vi "MALT Get Counter.vi"(8 "error in":errorcluster, 9 "Port":i32=1, 10 "Address":i32=3, 11 "FamilyCode":T1=enum."MALT132") -> (0 "error out":errorcluster, 3 "Value":u32)   [LabVIEW 2018, in "AltonTech MALT200817.lvlib"]
uses:
  <instrlib>/AltonTech MALT/AltonTech MALT200817.lvlib
  <instrlib>/AltonTech MALT/Public/Types/MALT CardTypes.ctl
  <instrlib>/AltonTech MALT/Private/Global/MALT Global.vi
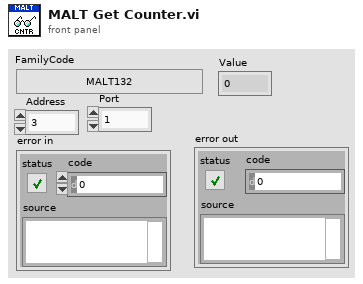
[diagram p1: front panel]
types:
  T1 = typedef "AltonTech MALT200817.lvlib/MALT CardTypes.ctl" = enum32{"-", "YAV90832", "YAV904X8", "MALT132", "YAV91616", "YAV90PIN", "YAV90096", "YAV90HVT", "YAV90CLR", "YAV90128", "YAV90PNE", "YAVCANCON", "YAV91775", "YAV90XXX", "YAV90MMU", "H730050", "H710060", "H710061", "YAV90304", "MMI", "YAV90060", "MALT160T", "YAV90059", "Not Defined"}
  T2 = cluster{"Timeout":i32, "CAN Response Delay":i32, "Connection ID":refnum<k5>}
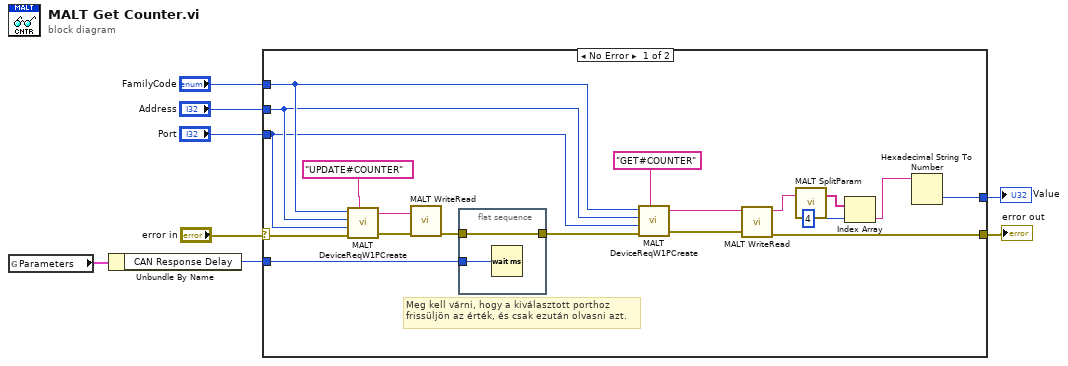
[diagram p0: block diagram]
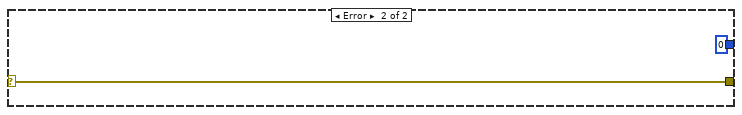
[diagram p2: hidden frame]
diagram:
  n1 = global read "MALT Global.vi" "Parameters"() -> (w3:T2)
  n2 = Unbundle By Name(w3) -> ("CAN Response Delay"=w2:i32)
  n3 = case shown="No Error" "error in" {
    selector: "error in" -> [w9 w31]
    tunnel: "FamilyCode" -> [w23 _]
    tunnel: "Address" -> [w22 _]
    tunnel: "Port" -> [w21 _]
    tunnel: [w12 w31] -> w5
    tunnel: [w11 u32 0] -> w4
    tunnel: w2 -> [w10 _]
    frame No Error {
      # "Meg kell várni, hogy a kiválasztott porthoz \nfrissüljön az érték, és csak ezután olvasni azt."
      n4 = call <instrlib>:"MALT DeviceReqW1PCreate.vi"("FamilyCode"=w23, "Address"=w22, "Param1"=w21, "error in"=w9, "Cmd"="UPDATE#COUNTER") -> ("Request"=w25:string, "error out"=w26:errorcluster)  [unwired: 1 in]
      n5 = call <instrlib>:"MALT WriteRead.vi"("error in"=w26, "Request"=w25) -> ("error out"=w19:errorcluster)  [unwired: 8 in, 1 out]
      n6 = flat-sequence {
        tunnel: [w29] -> w20
        tunnel: w19 -> [w29]
        tunnel: w10 -> [w28]
        frame #0 {
          n7 = Wait (ms)(milliseconds to wait=w28) -> ()  [unwired: 1 out]
        }
      }
      n8 = call <instrlib>:"MALT DeviceReqW1PCreate.vi"("FamilyCode"=w23, "Address"=w22, "Param1"=w21, "error in"=w20, "Cmd"="GET#COUNTER") -> ("Request"=w13:string, "error out"=w14:errorcluster)  [unwired: 1 in]
      n9 = call <instrlib>:"MALT WriteRead.vi"("error in"=w14, "Request"=w13) -> ("error out"=w12:errorcluster, "Response"=w17:string)  [unwired: 8 in]
      n10 = call <instrlib>:"MALT SplitParam.vi"("Line"=w17) -> ("Items"=w16:string[])  [unwired: 2 in]
      n11 = Index Array(array=w16, index=4) -> (element=w18:string)
      n12 = Hexadecimal String To Number(string=w18) -> (number=w11:u32)  [unwired: 2 in, 1 out]
    }
    frame Error {
    }
  }
  "error out" <- w5
  "Value" <- w4
